vi "Parameter Setup.vi"(7 "Row add 1":bool, 8 "Y direction total length- Height (um)":dbl, 9 "X direction total length- Width (um)":dbl, 10 "Quantity of Pixels of one step":dbl, 11 "Size of a single pixel (um)":dbl) -> (0 "Length of each Step (um)":i32, 2 "Number of Volumns":i32, 3 "Number of Rows":i32)   [LabVIEW 2015]
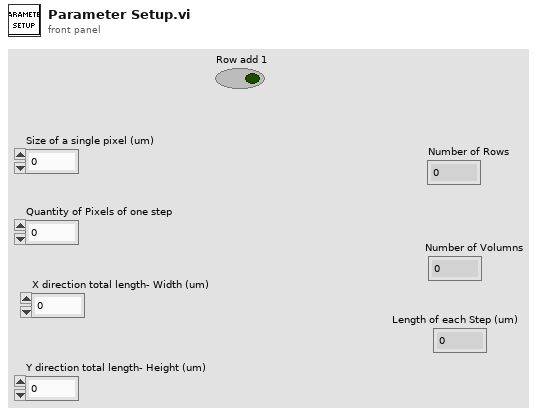
[diagram p1: front panel]
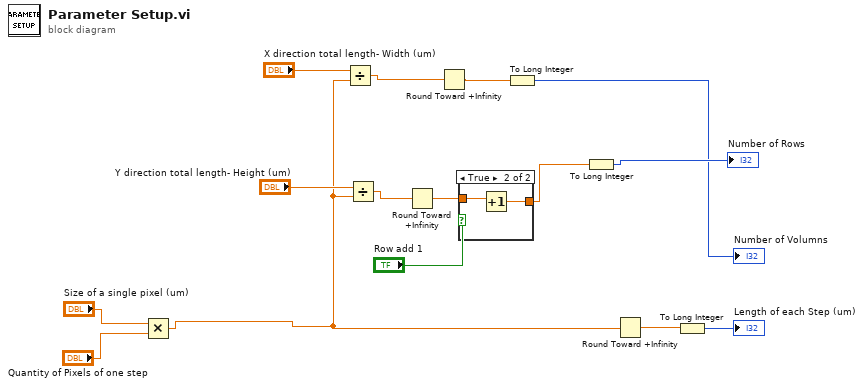
[diagram p0: block diagram]
diagram:
  n1 = Multiply(x="Size of a single pixel (um)", y="Quantity of Pixels of one step") -> (x*y=w8:dbl)
  n2 = Divide(x="X direction total length- Width (um)", y=w8) -> (x/y=w6:dbl)
  n3 = Divide(x="Y direction total length- Height (um)", y=w8) -> (x/y=w4:dbl)
  n4 = Round Toward +Infinity(x=w4) -> (ceil(x): smallest int >= x=w2:dbl)
  n5 = Round Toward +Infinity(x=w6) -> (ceil(x): smallest int >= x=w5:dbl)
  n6 = case shown="True" "Row add 1" {
    tunnel: [w16 w18] -> w3
    tunnel: w2 -> [w16 w17]
    frame False {
    }
    frame True {
      n7 = Increment(x=w17) -> (x+1=w18:dbl)
    }
  }
  n8 = To Long Integer(number=w5) -> (32bit integer=→"Number of Volumns":i32)
  n9 = To Long Integer(number=w3) -> (32bit integer=→"Number of Rows":i32)
  n10 = Round Toward +Infinity(x=w8) -> (ceil(x): smallest int >= x=w7:dbl)
  n11 = To Long Integer(number=w7) -> (32bit integer=→"Length of each Step (um)":i32)
